vi "ADS1115 (Backup).vi"() -> ()   [LabVIEW 2024]
uses:
  <vilib>/MakerHub/LINX/Private/Local IO/LinxI2cWrite.vi
  <vilib>/MakerHub/LINX/Public/Utilities/Check Channel.vi
  <vilib>/MakerHub/LINX/Private/Local IO/Handle Errors.vi
  <vilib>/MakerHub/LINX/Public/Utilities/Open Local.vi
  <vilib>/MakerHub/LINX/Private/Utilties/Generate Error.vi
  <vilib>/MakerHub/LINX/LMH-LINX.lvlib
panel:
  out "Channel 4":dbl format="%#.3f"
  in  "Channel 4":bool
  out "Channel 3":dbl format="%#.3f"
  in  "Channel 3":bool
  out "Channel 2":dbl format="%#.3f"
  in  "Channel 2":bool
  in  "Channel 1":bool
  in  "Conversion Mode":enum16{"One Channel", "Multiple Channel"}(ring)
  in  "Input Multiplexer (MUX)":u16(ring)=16384 items=["AIN0 - AIN1"=0, "AIN0 - AIN3"=4096, "AIN1 - AIN3"=8192, "AIN2 - AIN3"=12288, "AIN0 - GND"=16384, "AIN1 - GND"=20480, "AIN2 - GND"=24576, "AIN3 - GND"=28672]
  out "Channel 1":dbl format="%#.3f"
  out "Base Config":u16 format="%x"
  in  "Comparator Mode":u16(ring)=16 items=["Traditional"=0, "Window Comparator"=16]
  in  "Comparator Latch":u16(ring)=4 items=["Non-Latching"=0, "Latching"=4]
  in  "Comparator Polarity":u16(ring)=8 items=["Active Low"=0, "Active High"=8]
  in  "Comparator Queue":u16(ring)=3 items=["1 Conversion", "2 Conversions", "4 Conversions", "Disable Comparator"]
  in  "Data Rate":u16(ring)=224 items=["8 S/s"=0, "16 S/s"=32, "32 S/s"=64, "64 S/s"=96, "128 S/s"=128, "250 S/s"=160, "475 S/s"=192, "860 S/s"=224]
  in  "Mode Configuration":u16(ring) items=["Continuous Conversion"=0, "Single-Shot"=256]
  in  "Programmable Gain Amplifier (PGA)":u16(ring)=512 items=["±6.144 V"=0, "±4.096 V"=512, "±2.048 V"=1024, "±1.024 V"=1536, "±0.512 V"=2048, "±0.256 V"=2560, "±0.256 V"=3072, "±0.256 V"=3584]
  in  "Operational Status (OS)":u16(ring)=32768 items=["No Start"=0, "Start Conversion"=32768]
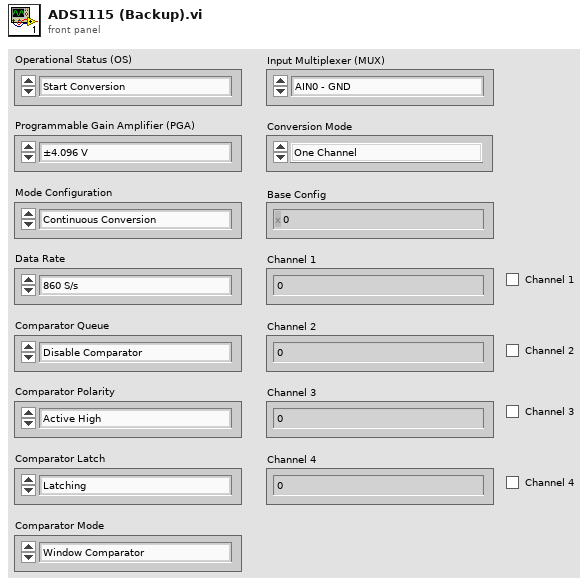
[diagram p1: front panel]
types:
  T1 = cluster{"I2C Slave Address":u8, "I2C Channel":u8}
  T2 = typedef "LMH-LINX.lvlib/LINX Ref.ctl" = cluster{"IO":T3, "Interface":T4, "LINX Device Config":T5}
  T3 = typedef "LMH-LINX.lvlib/Platform.ctl" = enum16{"Remote", "Local"}
  T4 = typedef "LMH-LINX.lvlib/Interface.ctl" = enum16{"Serial", "TCP"}
  T5 = typedef "LMH-LINX.lvlib/Device.lvlib/LINX Device Config.ctl" = cluster{"Interface":T4, "COM Port":refnum<visa-resource-name>, "TCP Configuration":T6, "Device Family":u8, "Device ID":u8, "Device Name":string, "TCP Ref":refnum<k5>, "Channels":T7}
  T6 = typedef "LMH-LINX.lvlib/Device.lvlib/TCP Config.ctl" = cluster{"IP Address":string, "Port":u16}
  T7 = typedef "LMH-LINX.lvlib/Channels.ctl" = cluster{"DI":u8[], "DO":u8[], "AI":u8[], "AO":u8[], "PWM":u8[], "QE":u8[], "UART":u8[], "I2C 2":u8[], "SPI":u8[], "CAN":u8[], "Servo":u8[], "AI Ref (V)":dbl, "AI Resolution (Bits)":u8, "AO Ref (V)":dbl, "AO Resolution (Bits)":u8}
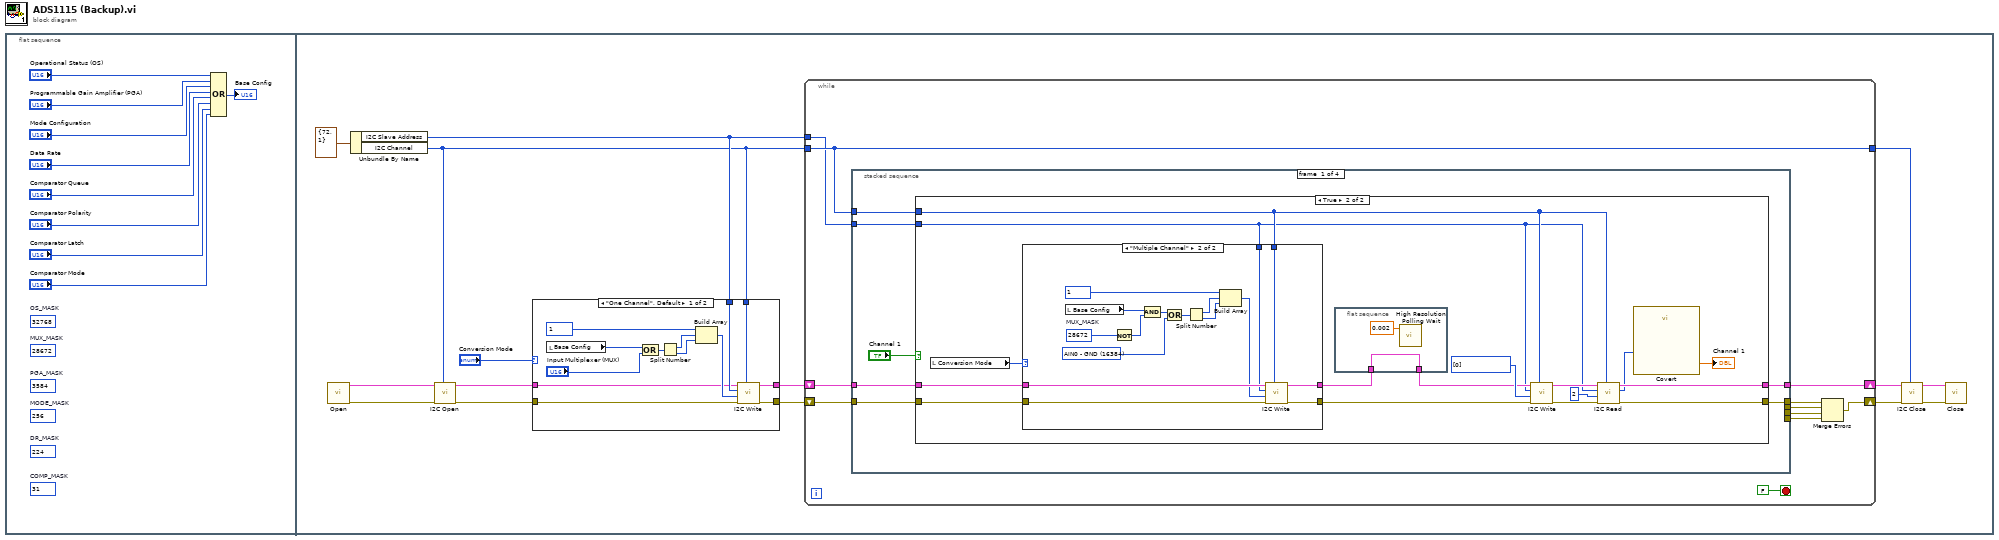
[diagram p0: block diagram]
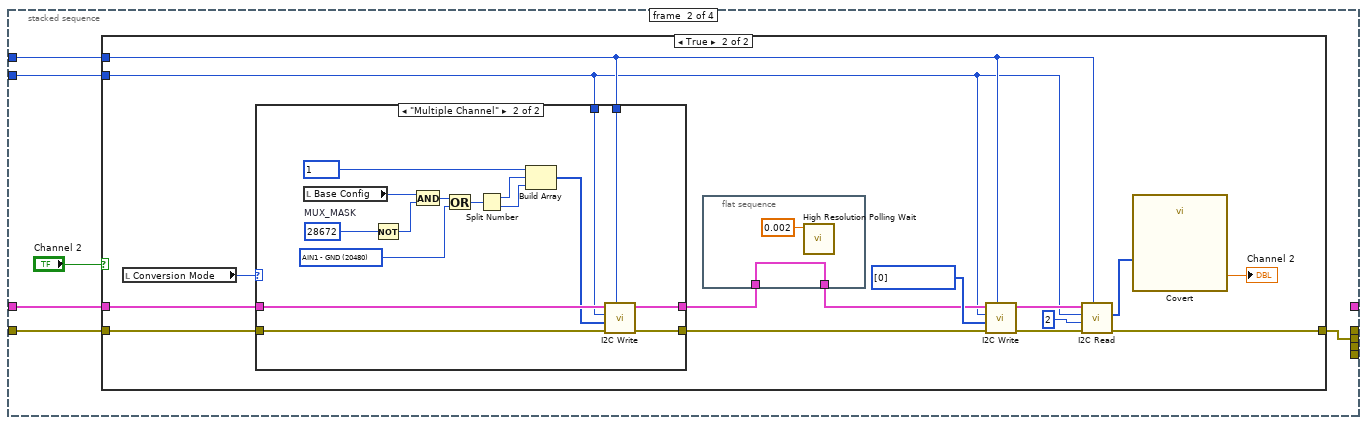
[diagram p5: hidden frame]
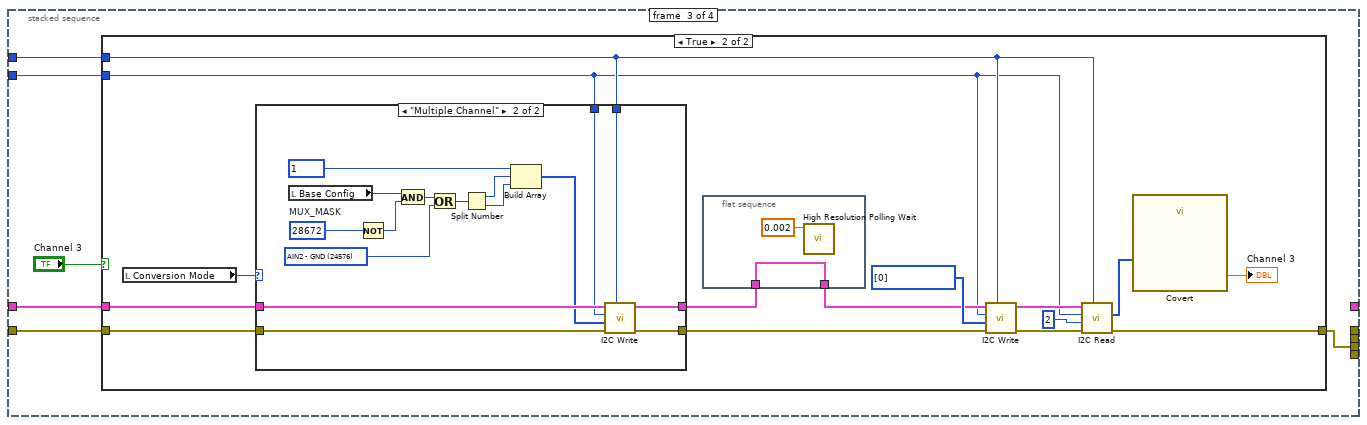
[diagram p8: hidden frame]
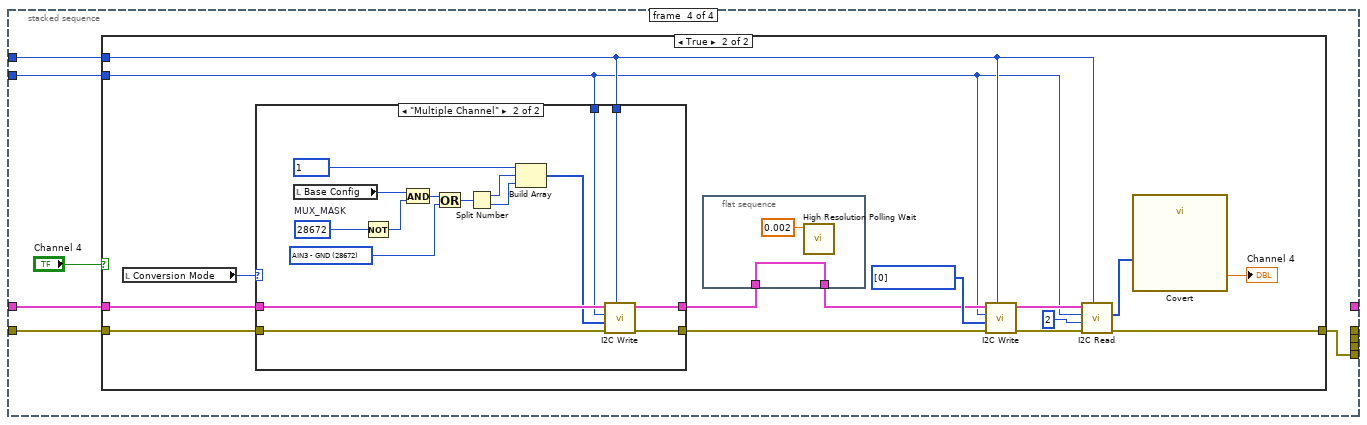
[diagram p11: hidden frame]
diagram:
  n1 = flat-sequence {
    frame #0 {
      (unwired) 31  # COMP_MASK
      (unwired) 224  # DR_MASK
      (unwired) 256  # MODE_MASK
      (unwired) 3584  # PGA_MASK
      (unwired) 28672  # MUX_MASK
      (unwired) 32768  # OS_MASK
      n2 = Compound Arithmetic op=OR("Operational Status (OS)", "Programmable Gain Amplifier (PGA)", "Mode Configuration", "Data Rate", "Comparator Queue", "Comparator Polarity", "Comparator Latch", "Comparator Mode") -> (→"Base Config":u16)
    }
    frame #1 {
      n3 = call-poly <vilib>:"Open.vi"() -> ("Error Out"=w15:errorcluster, "LINX Resource"=w23:T2)  [unwired: 9 in, 1 out]
      n4 = Unbundle By Name(T1 {"I2C Slave Address"=72, "I2C Channel"=1} ("Cluster")) -> ("I2C Slave Address"=w20:u8, "I2C Channel"=w11:u8)
      n5 = call <vilib>:"I2C Open.vi"("I2C Channel (0)"=w11, "Error In"=w15, "LINX Resource"=w23) -> ("Error Out"=w14:errorcluster, "LINX Resource"=w19:T2)  [unwired: 7 in]
      n6 = case shown="\"One Channel\", Default" "Conversion Mode" {
        tunnel: [w33 w38] -> w21
        tunnel: w20 -> [w32 _]
        tunnel: w19 -> [w31 w39]
        tunnel: w11 -> [w30 _]
        tunnel: w14 -> [w29 w38]
        tunnel: [w28 w39] -> w13
        frame "One Channel", Default {
          n7 = local read "Base Config"() -> (w37:u16)
          n8 = Compound Arithmetic op=OR(w37, "Input Multiplexer (MUX)") -> (w27:u16)
          n9 = Split Number(x=w27) -> (hi(x)=w26:u8, lo(x)=w25:u8)
          n10 = Build Array(1, w26, w25) -> (w35:i32[])
          n11 = call <vilib>:"I2C Write.vi"("I2C Channel"=w30, "Error In"=w29, "Data"=w35, "I2C Slave Address (0)"=w32, "LINX Resource"=w31) -> ("Error Out"=w33:errorcluster, "LINX Resource"=w28:T2)  [unwired: 5 in]
        }
        frame "Multiple Channel" {
        }
      }
      n12 = while {
        tunnel: w20 -> [w45]
        tunnel: w11 -> [w46]
        shift-right: [w50] -> w22
        shift-left: w13 -> [w49]
        shift-right: [w43] -> w17
        shift-left: w21 -> [w48]
        tunnel: [w46] -> w10
        stop <- FALSE stop-if-true
        n13 = stacked-sequence {
          tunnel: [w57 _ _ _] -> w50
          tunnel: w49 -> [w56 w101 w143 w185]
          tunnel: w48 -> [w55 w100 w142 w184]
          tunnel: [w54 _ _ _] -> w44
          tunnel: w46 -> [w53 w99 w141 w183]
          tunnel: w45 -> [w52 w98 w140 w182]
          tunnel: [_ w96 _ _] -> w42
          tunnel: [_ _ w138 _] -> w41
          tunnel: [_ _ _ w180] -> w40
          frame #0 {
            n14 = case shown="True" "Channel 1" {
              tunnel: [w59 w75] -> w57
              tunnel: w56 -> [w59 w65]
              tunnel: w55 -> [w58 w63]
              tunnel: [w58 w68] -> w54
              tunnel: w52 -> [_ w60]
              tunnel: w53 -> [_ w61]
              frame False {
              }
              frame True {
                n15 = local read "Conversion Mode"() -> (w62:enum16{"One Channel", "Multiple Channel"})
                n16 = case shown="\"Multiple Channel\"" w62 {
                  tunnel: [w77 w85] -> w66
                  tunnel: w65 -> [w77 w87]
                  tunnel: [w76 w84] -> w64
                  tunnel: w63 -> [w76 w86]
                  tunnel: w61 -> [_ w82]
                  tunnel: w60 -> [_ w81]
                  frame "One Channel", Default {
                  }
                  frame "Multiple Channel" {
                    w89 = u16 16384 items=["AIN0 - AIN1"=0, "AIN0 - AIN3"=4096, "AIN1 - AIN3"=8192, "AIN2 - AIN3"=12288, "AIN0 - GND"=16384, "AIN1 - GND"=20480, "AIN2 - GND"=24576, "AIN3 - GND"=28672] ("Input Multiplexer (MUX) 2")
                    w92 = u16 28672  # MUX_MASK
                    n17 = local read "Base Config"() -> (w93:u16)
                    n18 = Not(x=w92) -> (.not. x?=w91:u16)
                    n19 = And(x=w93, y=w91) -> (x .and. y?=w90:u16)
                    n20 = Or(x=w90, y=w89) -> (x .or. y?=w80:u16)
                    n21 = Split Number(x=w80) -> (hi(x)=w79:u8, lo(x)=w78:u8)
                    n22 = Build Array(1, w79, w78) -> (w83:i32[])
                    n23 = call <vilib>:"I2C Write.vi"("I2C Channel"=w82, "Error In"=w86, "Data"=w83, "I2C Slave Address (0)"=w81, "LINX Resource"=w87) -> ("Error Out"=w84:errorcluster, "LINX Resource"=w85:T2)  [unwired: 5 in]
                  }
                }
                n24 = flat-sequence {
                  tunnel: [w95] -> w67
                  tunnel: w66 -> [w95]
                  frame #0 {
                    n25 = call <vilib>:"High Resolution Polling Wait.vi"("seconds to wait"=0.002) -> ()  [unwired: 10 in, 1 out]
                  }
                }
                n26 = call <vilib>:"I2C Write.vi"("I2C Channel"=w61, "Error In"=w64, "Data"=i32[] [0], "I2C Slave Address (0)"=w60, "LINX Resource"=w67) -> ("Error Out"=w73:errorcluster, "LINX Resource"=w69:T2)  [unwired: 5 in]
                n27 = call <vilib>:"I2C Read.vi"("I2C Channel"=w61, "Error In"=w73, "Bytes To Read"=u8 2, "I2C Slave Address (0)"=w60, "LINX Resource"=w69) -> ("Error Out"=w68:errorcluster, "Data"=w71:u8[], "LINX Resource"=w75:T2)  [unwired: 4 in]
                n28 = call "Covert.vi"("Data"=w71) -> ("Value"=→"Channel 1":dbl)  [unwired: 10 in]
              }
            }
          }
          frame #1 {
            n29 = case shown="True" "Channel 2" {
              tunnel: w101 -> [_ w108]
              tunnel: w100 -> [w102 w106]
              tunnel: [w102 w111] -> w96
              tunnel: w98 -> [_ w103]
              tunnel: w99 -> [_ w104]
              frame False {
              }
              frame True {
                n30 = local read "Conversion Mode"() -> (w105:enum16{"One Channel", "Multiple Channel"})
                n31 = case shown="\"Multiple Channel\"" w105 {
                  tunnel: [w119 w133] -> w109
                  tunnel: w108 -> [w119 w135]
                  tunnel: [w118 w132] -> w107
                  tunnel: w106 -> [w118 w134]
                  tunnel: w104 -> [_ w131]
                  tunnel: w103 -> [_ w130]
                  frame "One Channel", Default {
                  }
                  frame "Multiple Channel" {
                    w125 = u16 20480 items=["AIN0 - AIN1"=0, "AIN0 - AIN3"=4096, "AIN1 - AIN3"=8192, "AIN2 - AIN3"=12288, "AIN0 - GND"=16384, "AIN1 - GND"=20480, "AIN2 - GND"=24576, "AIN3 - GND"=28672] ("Input Multiplexer (MUX) 2")
                    w128 = u16 28672  # MUX_MASK
                    n32 = local read "Base Config"() -> (w129:u16)
                    n33 = Not(x=w128) -> (.not. x?=w127:u16)
                    n34 = And(x=w129, y=w127) -> (x .and. y?=w126:u16)
                    n35 = Or(x=w126, y=w125) -> (x .or. y?=w123:u16)
                    n36 = Split Number(x=w123) -> (hi(x)=w122:u8, lo(x)=w121:u8)
                    n37 = Build Array(1, w122, w121) -> (w120:i32[])
                    n38 = call <vilib>:"I2C Write.vi"("I2C Channel"=w131, "Error In"=w134, "Data"=w120, "I2C Slave Address (0)"=w130, "LINX Resource"=w135) -> ("Error Out"=w132:errorcluster, "LINX Resource"=w133:T2)  [unwired: 5 in]
                  }
                }
                n39 = flat-sequence {
                  tunnel: [w136] -> w110
                  tunnel: w109 -> [w136]
                  frame #0 {
                    n40 = call <vilib>:"High Resolution Polling Wait.vi"("seconds to wait"=0.002) -> ()  [unwired: 10 in, 1 out]
                  }
                }
                n41 = call <vilib>:"I2C Write.vi"("I2C Channel"=w104, "Error In"=w107, "Data"=i32[] [0], "I2C Slave Address (0)"=w103, "LINX Resource"=w110) -> ("Error Out"=w116:errorcluster, "LINX Resource"=w112:T2)  [unwired: 5 in]
                n42 = call <vilib>:"I2C Read.vi"("I2C Channel"=w104, "Error In"=w116, "Bytes To Read"=u8 2, "I2C Slave Address (0)"=w103, "LINX Resource"=w112) -> ("Error Out"=w111:errorcluster, "Data"=w114:u8[])  [unwired: 4 in, 1 out]
                n43 = call "Covert.vi"("Data"=w114) -> ("Value"=→"Channel 2":dbl)  [unwired: 10 in]
              }
            }
          }
          frame #2 {
            n44 = case shown="True" "Channel 3" {
              tunnel: w143 -> [_ w150]
              tunnel: w142 -> [w144 w148]
              tunnel: [w144 w153] -> w138
              tunnel: w140 -> [_ w145]
              tunnel: w141 -> [_ w146]
              frame False {
              }
              frame True {
                n45 = local read "Conversion Mode"() -> (w147:enum16{"One Channel", "Multiple Channel"})
                n46 = case shown="\"Multiple Channel\"" w147 {
                  tunnel: [w161 w175] -> w151
                  tunnel: w150 -> [w161 w177]
                  tunnel: [w160 w174] -> w149
                  tunnel: w148 -> [w160 w176]
                  tunnel: w146 -> [_ w173]
                  tunnel: w145 -> [_ w172]
                  frame "One Channel", Default {
                  }
                  frame "Multiple Channel" {
                    w167 = u16 24576 items=["AIN0 - AIN1"=0, "AIN0 - AIN3"=4096, "AIN1 - AIN3"=8192, "AIN2 - AIN3"=12288, "AIN0 - GND"=16384, "AIN1 - GND"=20480, "AIN2 - GND"=24576, "AIN3 - GND"=28672] ("Input Multiplexer (MUX) 2")
                    w170 = u16 28672  # MUX_MASK
                    n47 = local read "Base Config"() -> (w171:u16)
                    n48 = Not(x=w170) -> (.not. x?=w169:u16)
                    n49 = And(x=w171, y=w169) -> (x .and. y?=w168:u16)
                    n50 = Or(x=w168, y=w167) -> (x .or. y?=w165:u16)
                    n51 = Split Number(x=w165) -> (hi(x)=w164:u8, lo(x)=w163:u8)
                    n52 = Build Array(1, w164, w163) -> (w162:i32[])
                    n53 = call <vilib>:"I2C Write.vi"("I2C Channel"=w173, "Error In"=w176, "Data"=w162, "I2C Slave Address (0)"=w172, "LINX Resource"=w177) -> ("Error Out"=w174:errorcluster, "LINX Resource"=w175:T2)  [unwired: 5 in]
                  }
                }
                n54 = flat-sequence {
                  tunnel: [w178] -> w152
                  tunnel: w151 -> [w178]
                  frame #0 {
                    n55 = call <vilib>:"High Resolution Polling Wait.vi"("seconds to wait"=0.002) -> ()  [unwired: 10 in, 1 out]
                  }
                }
                n56 = call <vilib>:"I2C Write.vi"("I2C Channel"=w146, "Error In"=w149, "Data"=i32[] [0], "I2C Slave Address (0)"=w145, "LINX Resource"=w152) -> ("Error Out"=w158:errorcluster, "LINX Resource"=w154:T2)  [unwired: 5 in]
                n57 = call <vilib>:"I2C Read.vi"("I2C Channel"=w146, "Error In"=w158, "Bytes To Read"=u8 2, "I2C Slave Address (0)"=w145, "LINX Resource"=w154) -> ("Error Out"=w153:errorcluster, "Data"=w156:u8[])  [unwired: 4 in, 1 out]
                n58 = call "Covert.vi"("Data"=w156) -> ("Value"=→"Channel 3":dbl)  [unwired: 10 in]
              }
            }
          }
          frame #3 {
            n59 = case shown="True" "Channel 4" {
              tunnel: w185 -> [_ w192]
              tunnel: w184 -> [w186 w190]
              tunnel: [w186 w195] -> w180
              tunnel: w182 -> [_ w187]
              tunnel: w183 -> [_ w188]
              frame False {
              }
              frame True {
                n60 = local read "Conversion Mode"() -> (w189:enum16{"One Channel", "Multiple Channel"})
                n61 = case shown="\"Multiple Channel\"" w189 {
                  tunnel: [w203 w217] -> w193
                  tunnel: w192 -> [w203 w219]
                  tunnel: [w202 w216] -> w191
                  tunnel: w190 -> [w202 w218]
                  tunnel: w188 -> [_ w215]
                  tunnel: w187 -> [_ w214]
                  frame "One Channel", Default {
                  }
                  frame "Multiple Channel" {
                    w206 = u16 28672 items=["AIN0 - AIN1"=0, "AIN0 - AIN3"=4096, "AIN1 - AIN3"=8192, "AIN2 - AIN3"=12288, "AIN0 - GND"=16384, "AIN1 - GND"=20480, "AIN2 - GND"=24576, "AIN3 - GND"=28672] ("Input Multiplexer (MUX) 2")
                    w205 = u16 28672  # MUX_MASK
                    n62 = local read "Base Config"() -> (w213:u16)
                    n63 = Not(x=w205) -> (.not. x?=w212:u16)
                    n64 = And(x=w213, y=w212) -> (x .and. y?=w211:u16)
                    n65 = Or(x=w211, y=w206) -> (x .or. y?=w210:u16)
                    n66 = Split Number(x=w210) -> (hi(x)=w209:u8, lo(x)=w208:u8)
                    n67 = Build Array(1, w209, w208) -> (w204:i32[])
                    n68 = call <vilib>:"I2C Write.vi"("I2C Channel"=w215, "Error In"=w218, "Data"=w204, "I2C Slave Address (0)"=w214, "LINX Resource"=w219) -> ("Error Out"=w216:errorcluster, "LINX Resource"=w217:T2)  [unwired: 5 in]
                  }
                }
                n69 = flat-sequence {
                  tunnel: [w220] -> w194
                  tunnel: w193 -> [w220]
                  frame #0 {
                    n70 = call <vilib>:"High Resolution Polling Wait.vi"("seconds to wait"=0.002) -> ()  [unwired: 10 in, 1 out]
                  }
                }
                n71 = call <vilib>:"I2C Write.vi"("I2C Channel"=w188, "Error In"=w191, "Data"=i32[] [0], "I2C Slave Address (0)"=w187, "LINX Resource"=w194) -> ("Error Out"=w200:errorcluster, "LINX Resource"=w196:T2)  [unwired: 5 in]
                n72 = call <vilib>:"I2C Read.vi"("I2C Channel"=w188, "Error In"=w200, "Bytes To Read"=u8 2, "I2C Slave Address (0)"=w187, "LINX Resource"=w196) -> ("Error Out"=w195:errorcluster, "Data"=w198:u8[])  [unwired: 4 in, 1 out]
                n73 = call "Covert.vi"("Data"=w198) -> ("Value"=→"Channel 4":dbl)  [unwired: 10 in]
              }
            }
          }
        }
        n74 = Merge Errors(w44, w42, w41, w40) -> (w43:errorcluster)
      }
      n75 = call <vilib>:"I2C Close.vi"("I2C Channel (0)"=w10, "Error In"=w17, "LINX Resource"=w22) -> ("Error Out"=w16:errorcluster, "LINX Resource"=w18:T2)  [unwired: 7 in]
      n76 = call <vilib>:"Close.vi"("Error In"=w16, "LINX Resource"=w18) -> ()  [unwired: 9 in, 1 out]
    }
  }
